vi "浊度电极校准.vi"() -> ()   [LabVIEW 2016, in "斯坦道多参数.lvlib"]
uses:
  <vilib>/Utility/miscctls.llb/LVPointTypeDef.ctl
  <vilib>/Utility/miscctls.llb/LVPositionTypeDef.ctl
  <vilib>/Analysis/NI_AALBase.lvlib
panel:
  in  "刷新按钮":bool
  out "第三点信号值":dbl
  out "第二点信号值":dbl
  out "第一点信号值":dbl
  out "温度":dbl format="%#.2f"
  out "通讯状态":string
  out "电极状态标志":u16(ring) items=["OK"=0, "第一点校正通过"=1, "第二点校正通过"=2, "悬浮物两点校准第一点校正通过"=11, "悬浮物两点校准第二点校正通过"=12, "浊度三点校正第一点校正通过"=31, "浊度三点校正第二点校正通过"=32, "浊度三点校正第三点校正通过"=33]
  out "第三点校准值":dbl
  out "标液3":dbl
  out "第二点校准值":dbl
  out "第一点校准值":dbl
  in  "校准停止":bool
  in  "校准启动":bool
  in  "校准模式":enum16{"两点校准", "单点校准", "三点校准"}(ring)
  out "最小值":sgl format="%#.2f"
  out "最大值":sgl format="%#.2f"
  out "波形图表":sgl(graph) caption="历史曲线"
  out "mean":dbl caption="均值" format="%#.2f"
  out "standard deviation":dbl caption="标准差" format="%#.2f"
  out "变异系数":dbl format="%#.6f"
  out "测量值":dbl format="%#.2f"
  out "提示":string
  out "标液2":dbl
  out "标液1":dbl
  out "信号值":dbl format="%#.2f"
  out "偏移值补偿":dbl caption="浊度偏移修正值" format="%#.2f"
  out "电极斜率":dbl format="%#.6f"
  out "电极零点":dbl format="%#.6f"
  # "浊度电极设定"
  # "℃"
  # "NTU"
  # "%"
  # "NTU"
  # "请选择校准模式:"
  # "NTU"
  # "NTU"
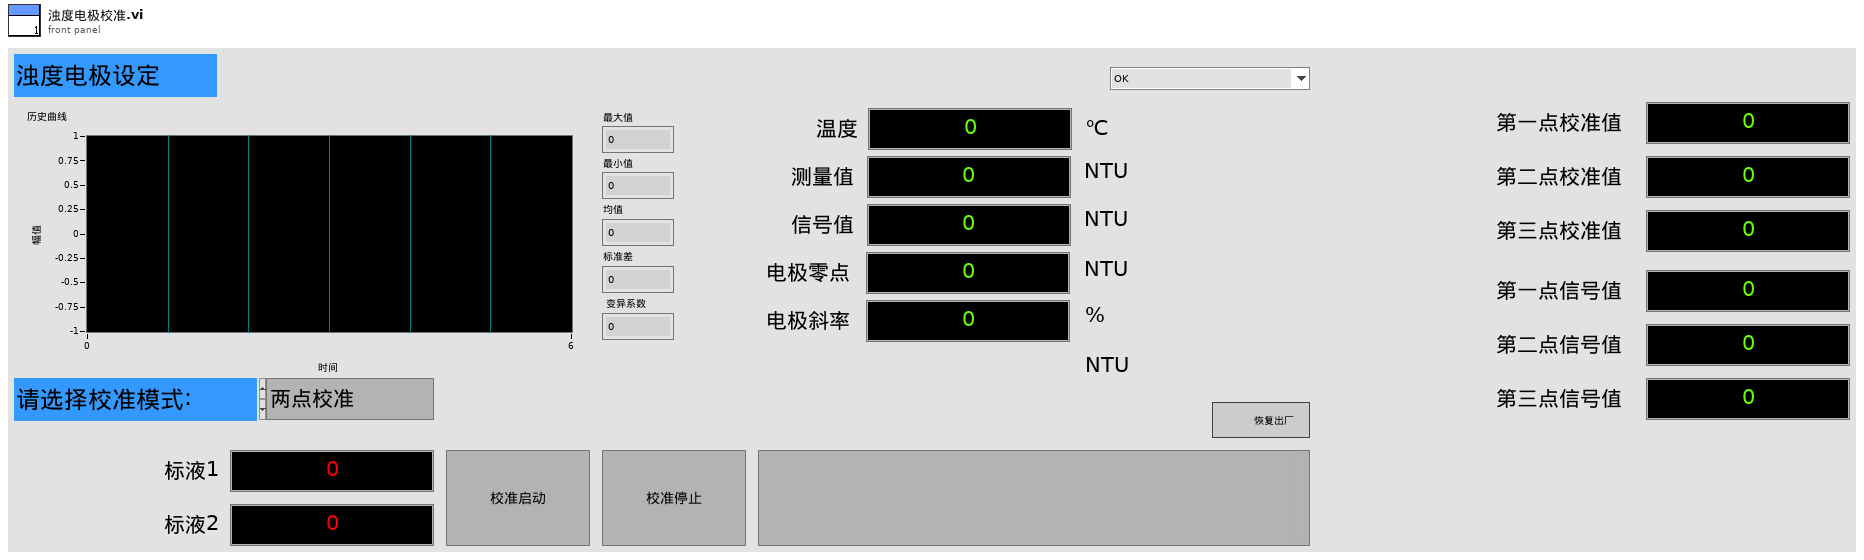
[diagram p1: front panel]
types:
  T1 = typedef "LVPointTypeDef.ctl" = cluster{"Horizontal":i16, "Vertical":i16}
  T2 = cluster{"电极状态标志":u16, "电极型号标志":u16, "浊度测量值":sgl, "温度测量值":sgl, "浊度信号值":sgl, "浊度偏移修正值":sgl, "温度偏移修正值":sgl, "手动温度补偿值":sgl, "浊度电极零点":sgl, "浊度电极斜率":sgl, "第1点标准值记录":sgl, "第1点信号值记录":sgl, "第1点温度值记录":sgl, "第2点标准值记录":sgl, "第2点信号值记录":sgl, "第2点温度值记录":sgl, "命令滤波设定":u16, "温度模式":enum16{"ATC", "MTC"}, "生产批次":u16, "电极序号":u16, "串口地址":u16, "串口波特率":enum16{"9600", "19200", "115200"}, "串口校验位":enum16{"NONE", "ODD", "EVEN"}, "串口停止位":enum16{"1bit", "2bit"}, "第一点标准值":sgl, "第二点标准值":sgl, "第三点标准值":sgl}
  T3 = typedef "LVPositionTypeDef.ctl" = cluster{"Left":i32, "Top":i32}
  T4 = enum8{"Enabled", "Disabled", "Disabled and Grayed Out"}
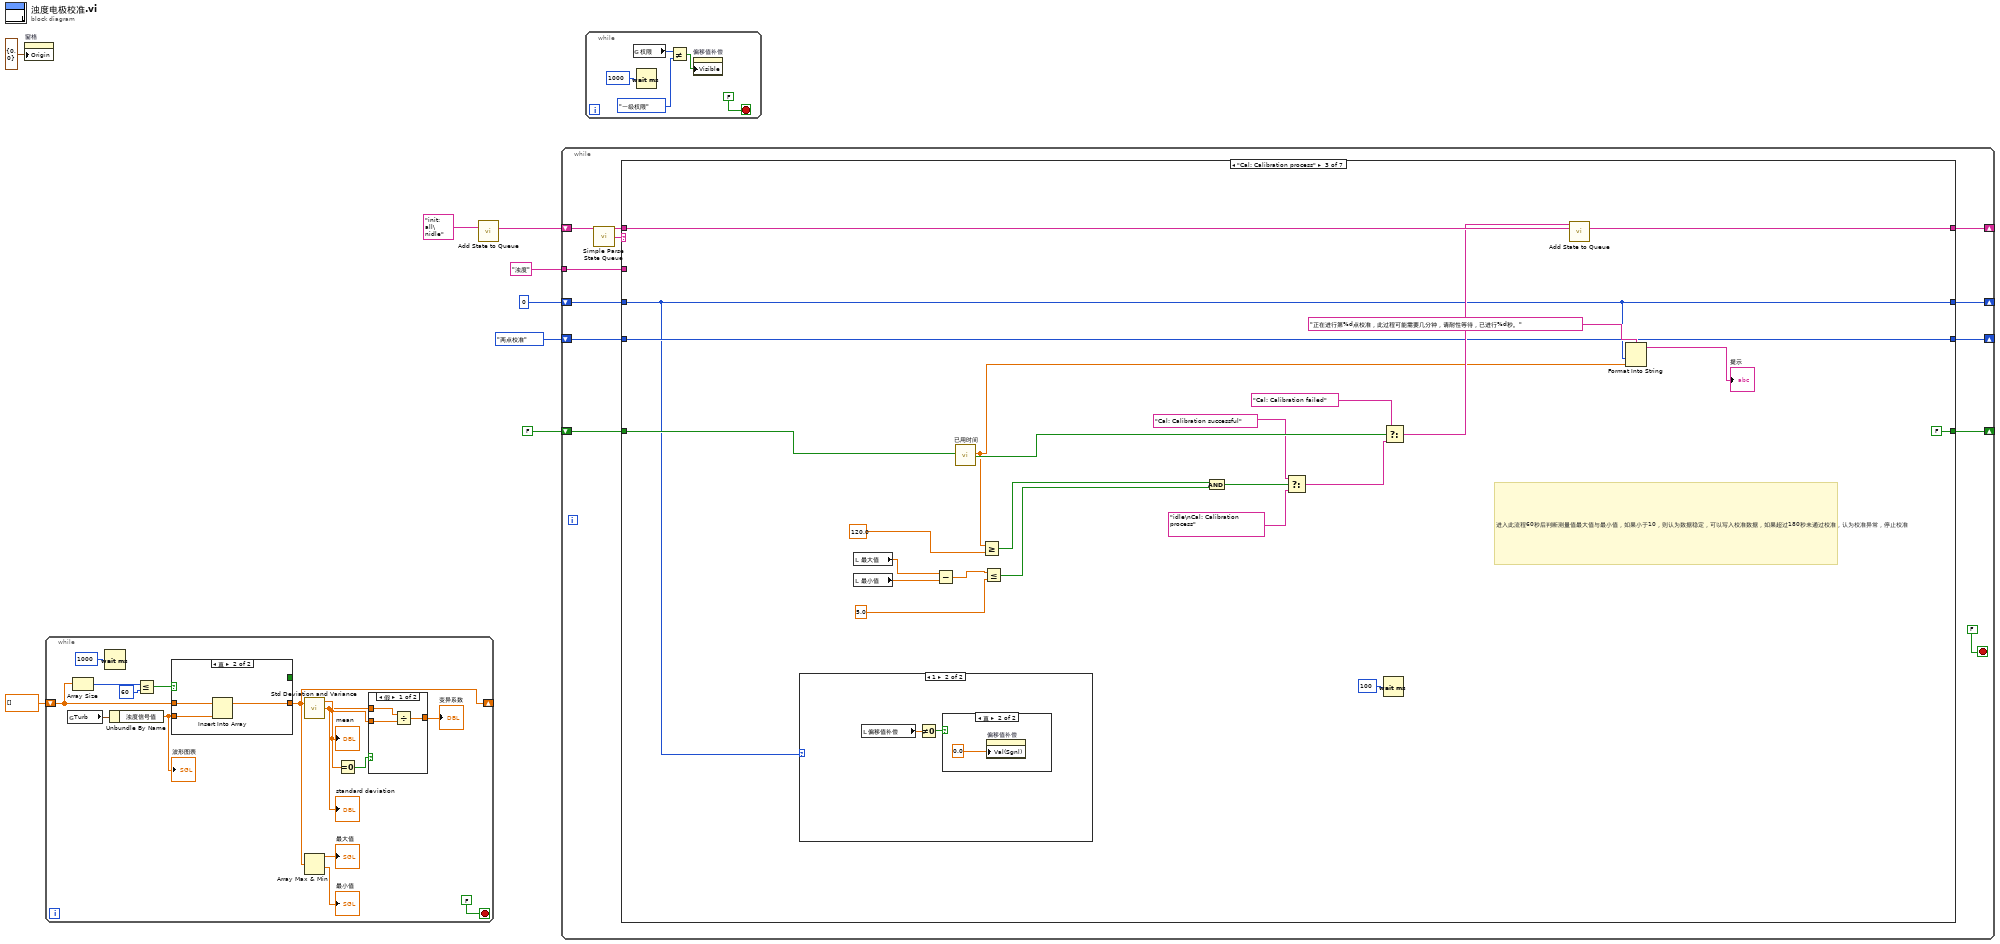
[diagram p0: block diagram]
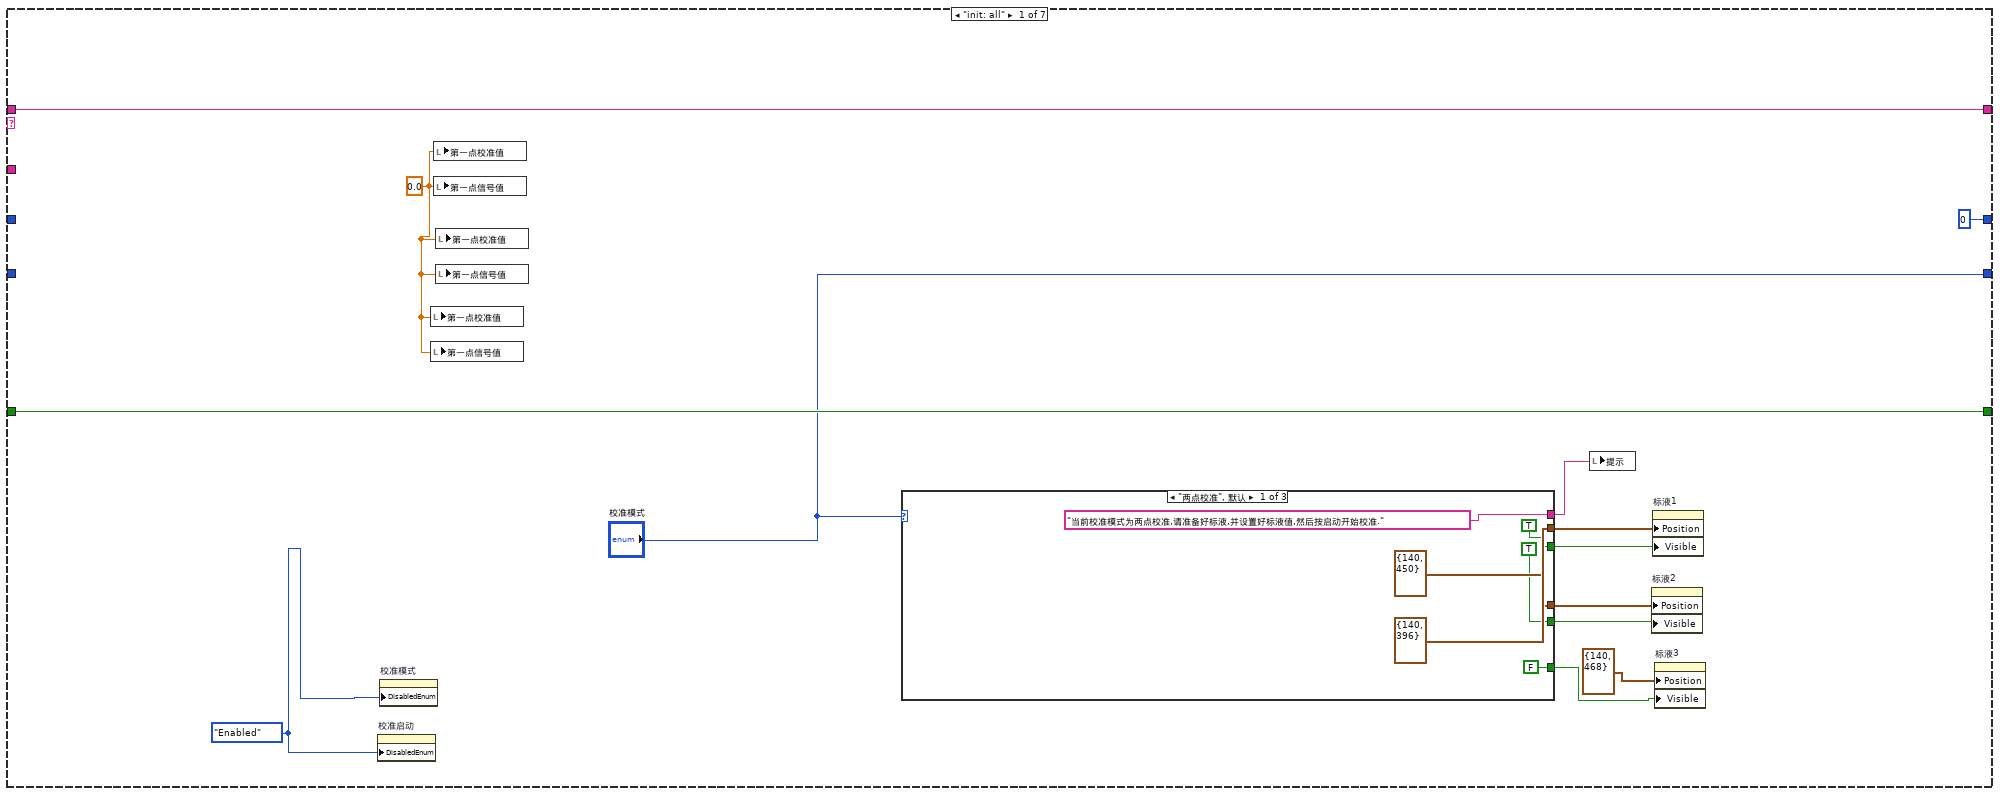
[diagram p2: hidden frame]
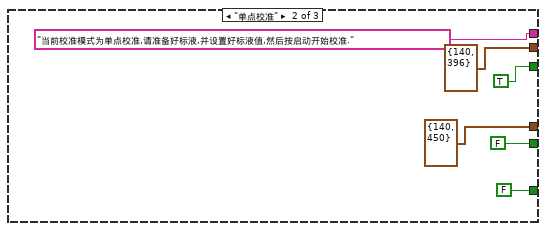
[diagram p3: hidden frame]
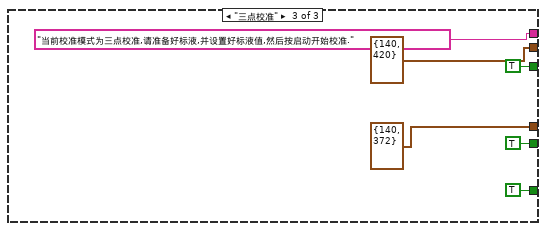
[diagram p4: hidden frame]
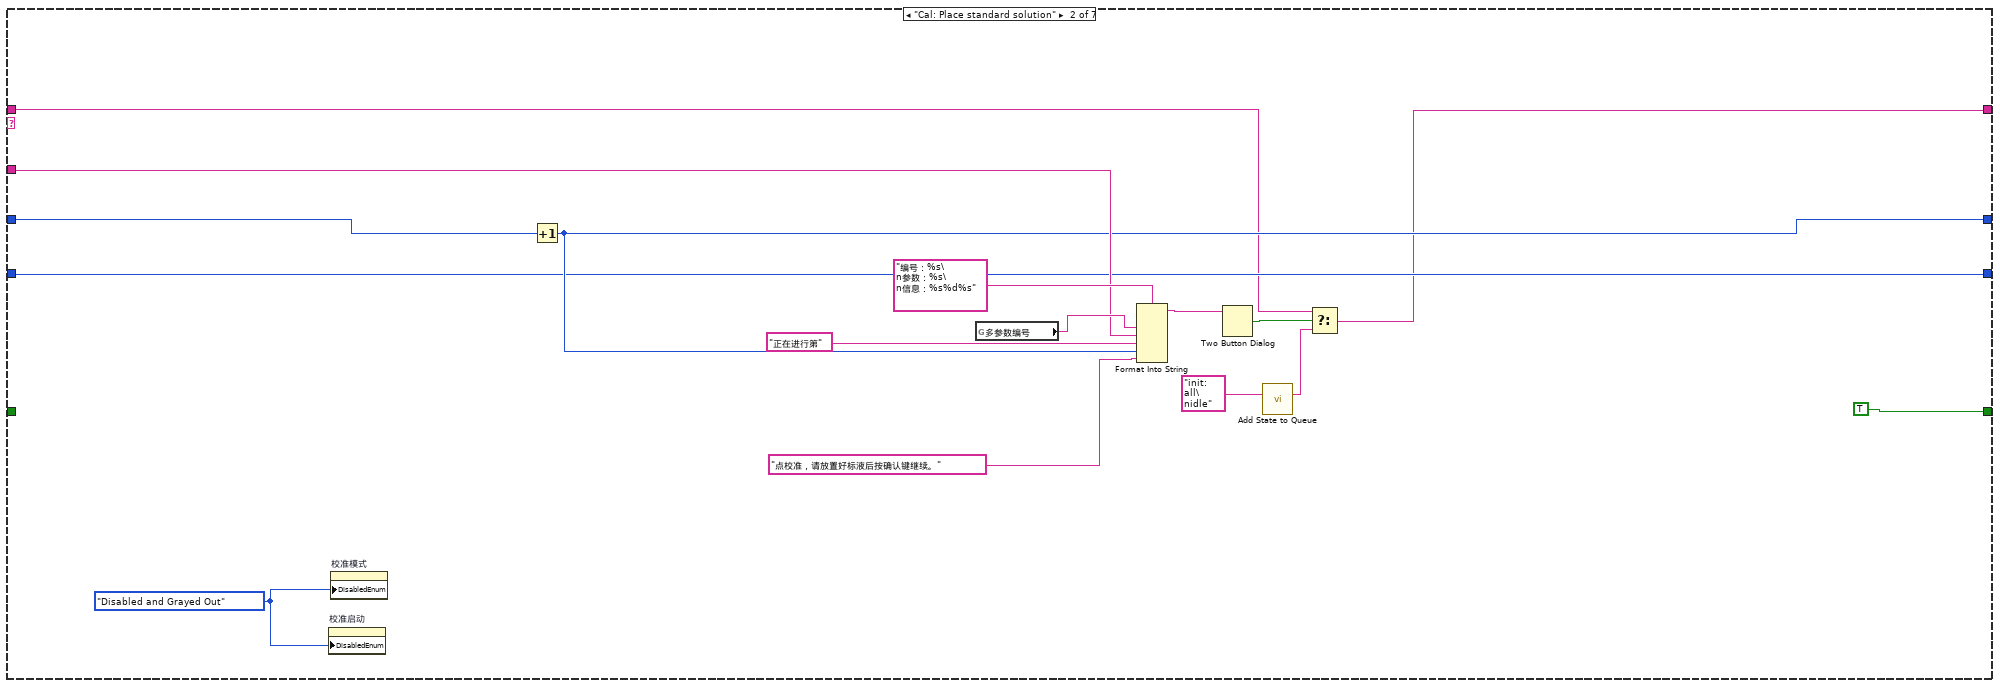
[diagram p5: hidden frame]
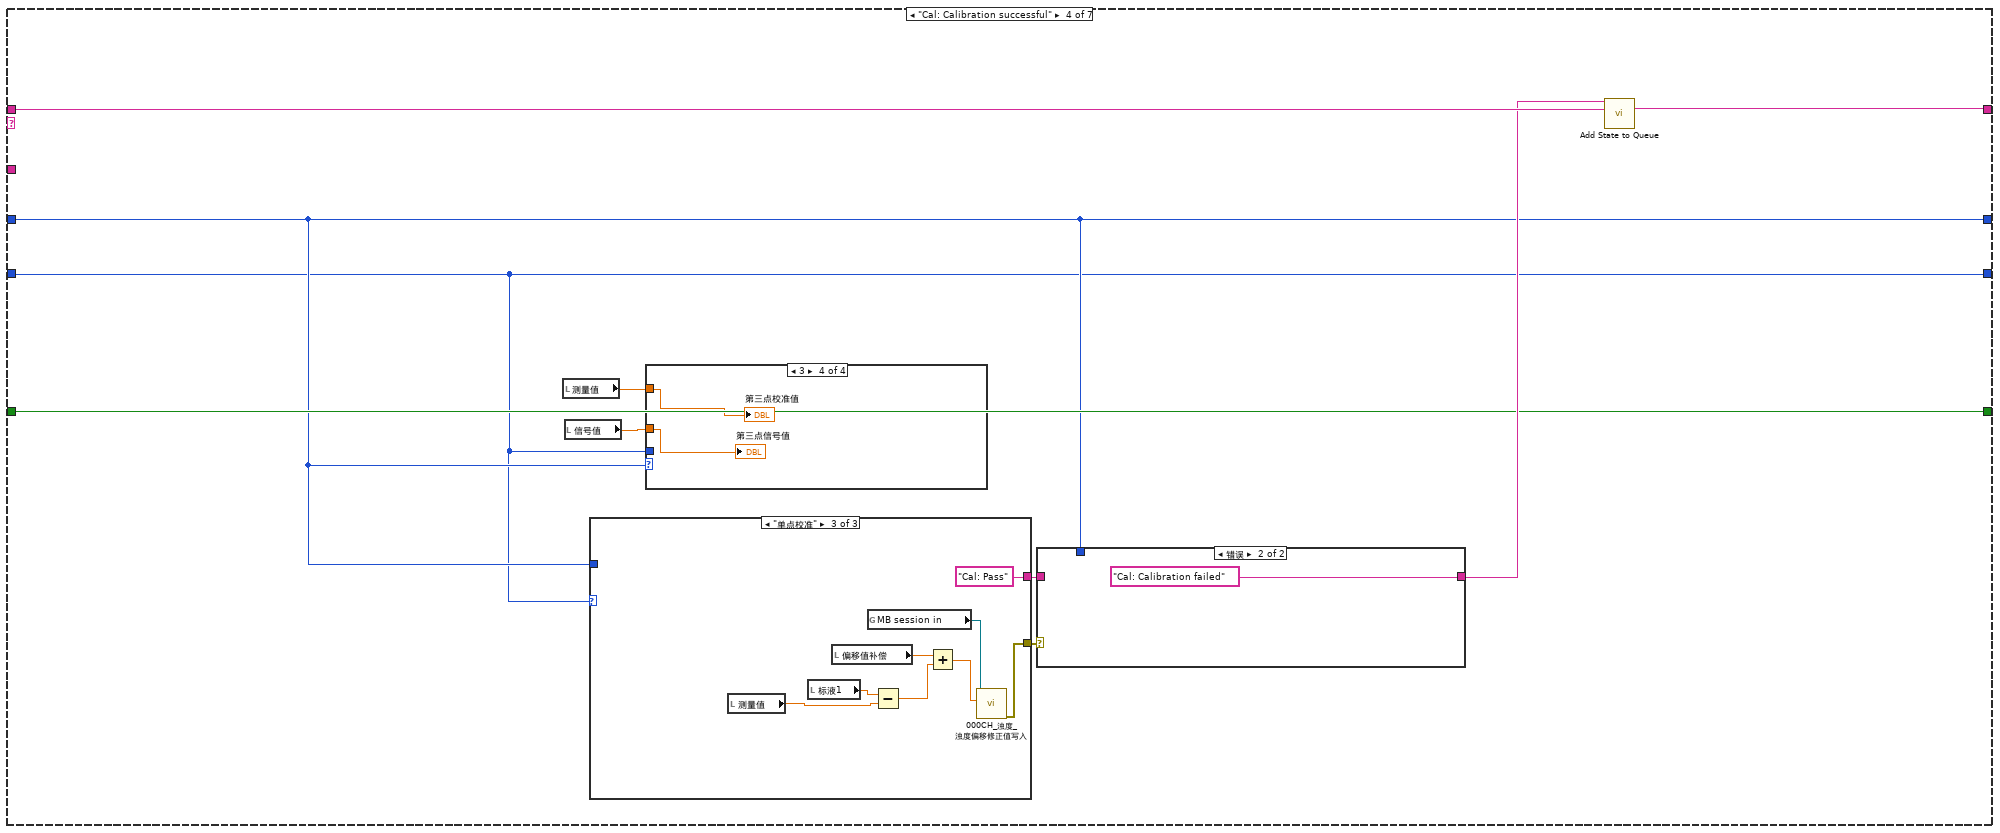
[diagram p8: hidden frame]
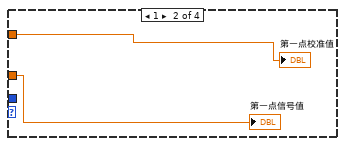
[diagram p10: hidden frame]
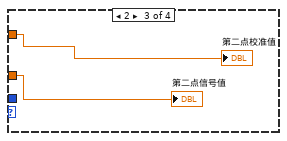
[diagram p11: hidden frame]
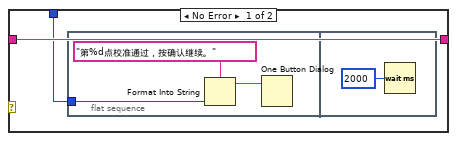
[diagram p12: hidden frame]
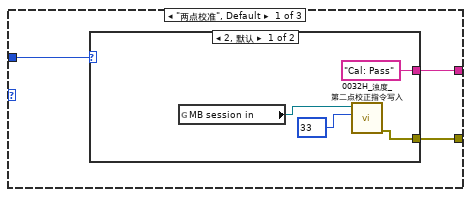
[diagram p13: hidden frame]
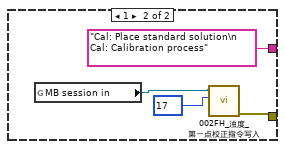
[diagram p14: hidden frame]
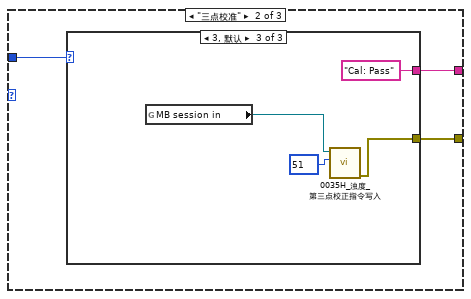
[diagram p15: hidden frame]
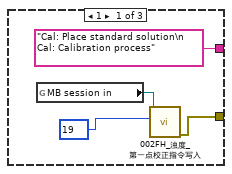
[diagram p16: hidden frame]
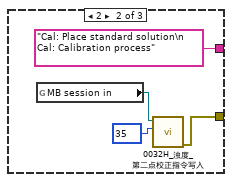
[diagram p17: hidden frame]
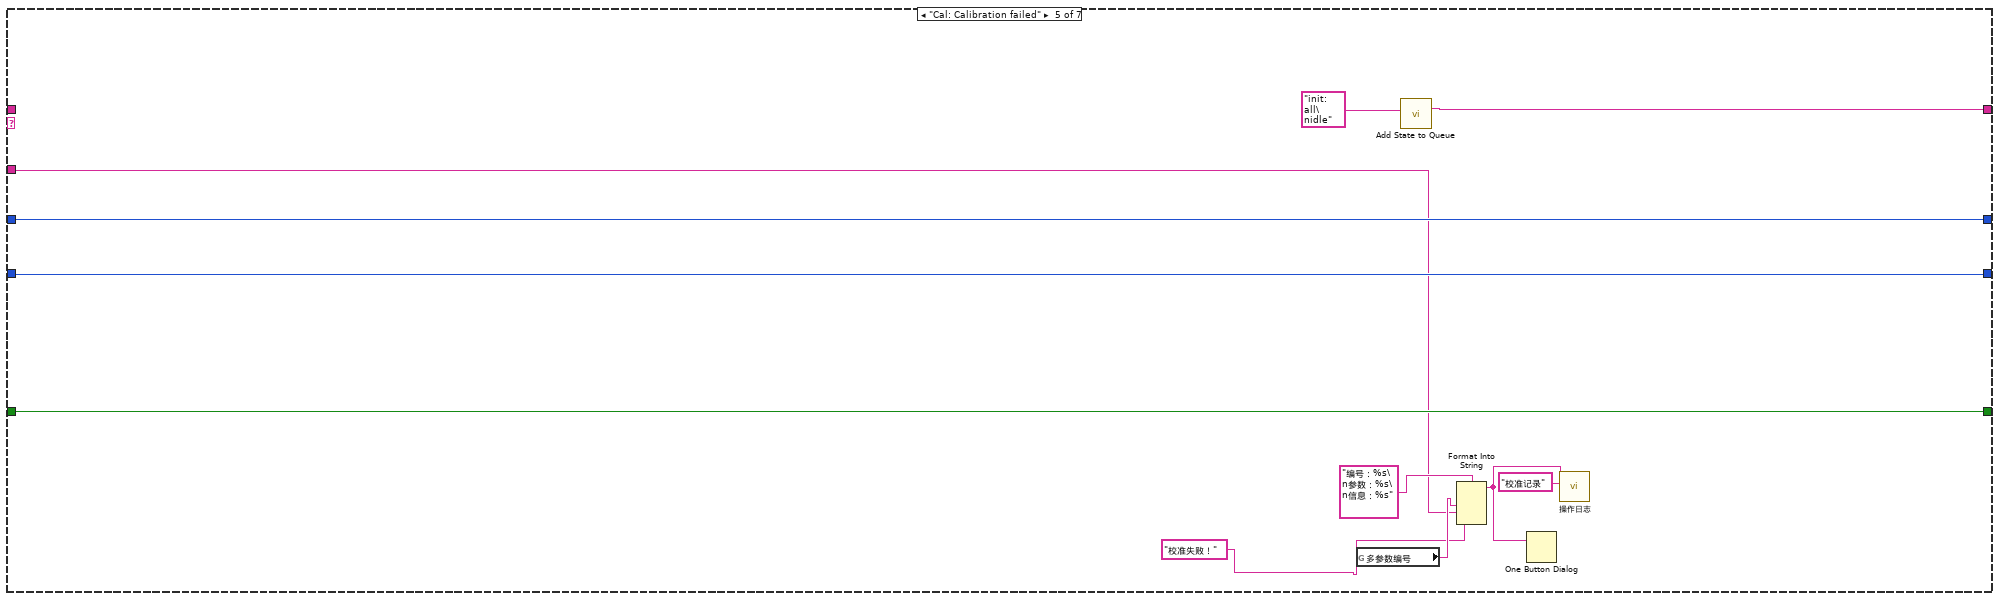
[diagram p18: hidden frame]
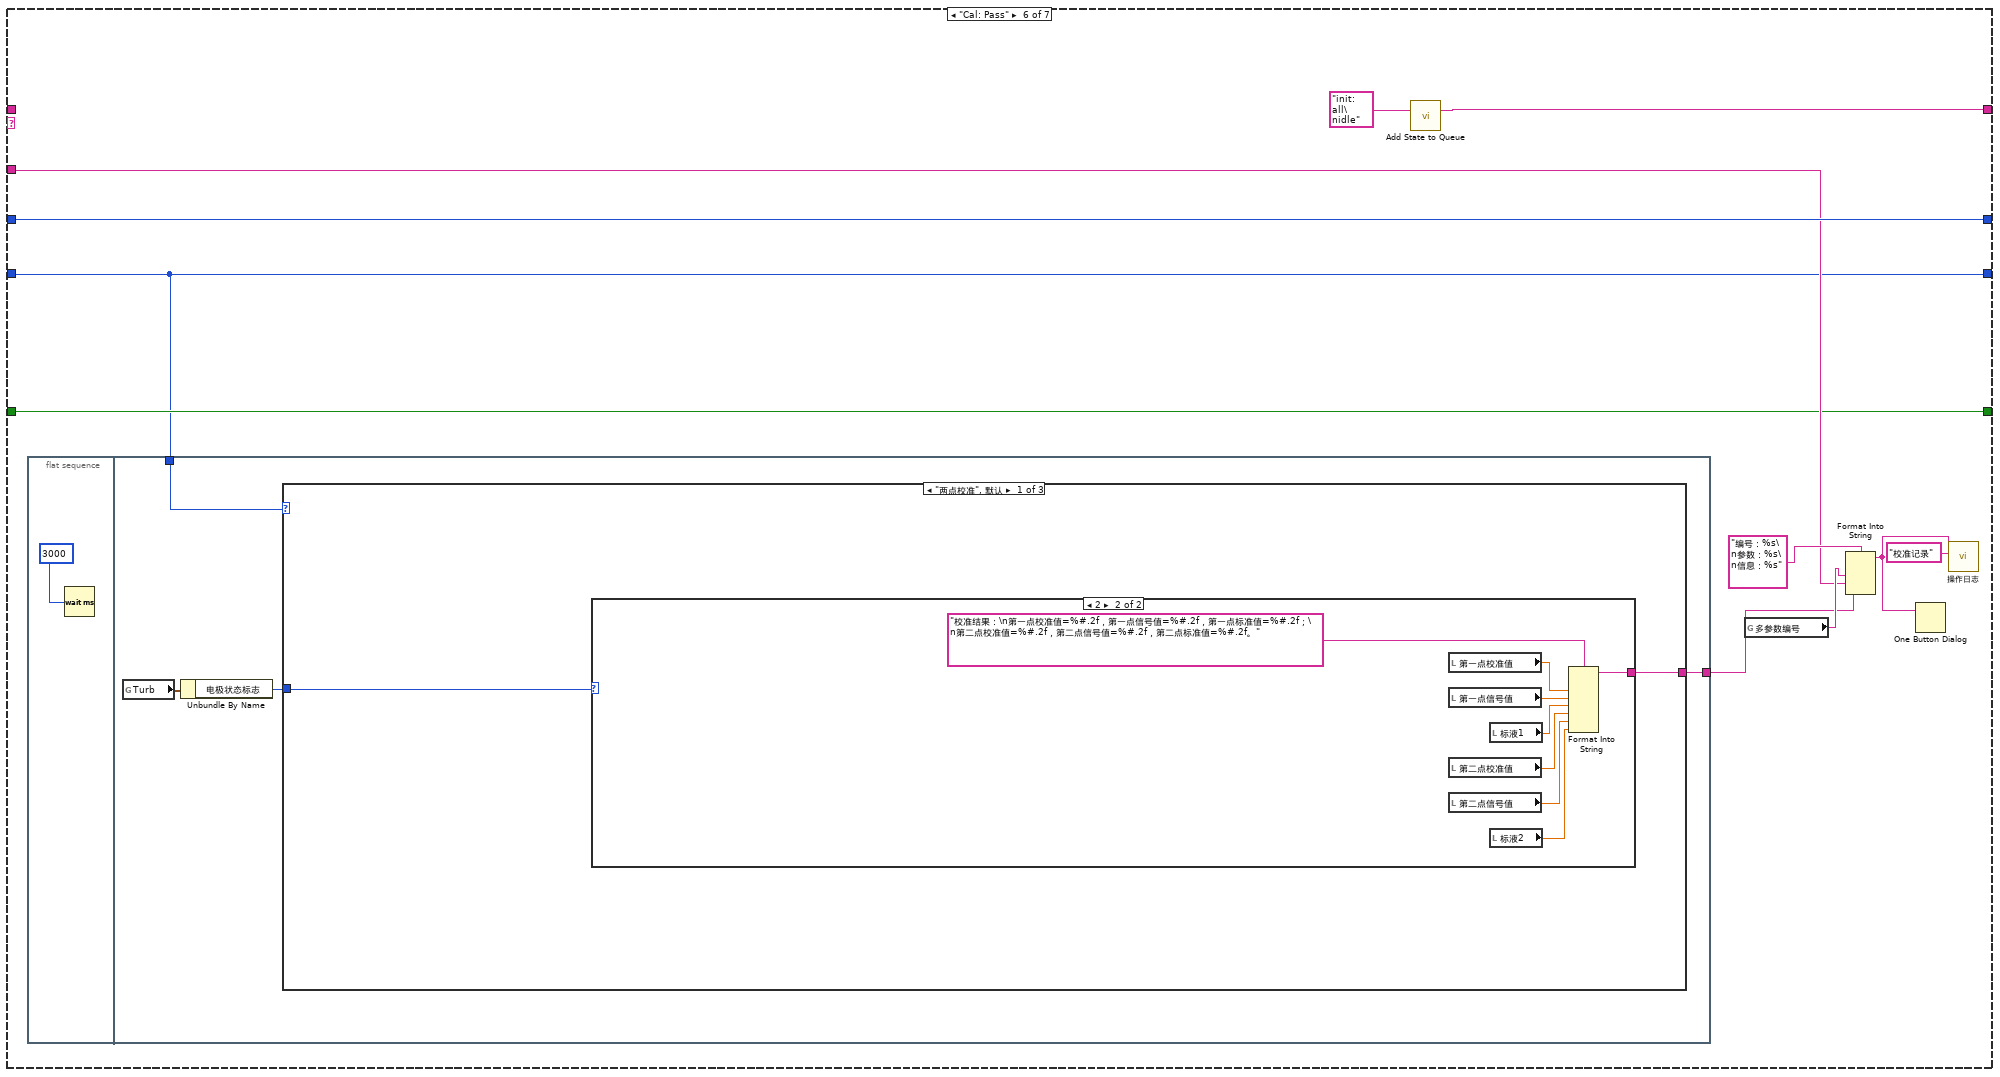
[diagram p19: hidden frame]
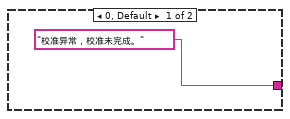
[diagram p20: hidden frame]
diagram:
  n1 = property on="窗格" class="Pane"("Origin"=T1 {"Horizontal"=0, "Vertical"=0} ("原点")) -> ()  [unwired: 2 in, 2 out]
  n2 = while {
    shift-right: [w12] -> _
    shift-left: sgl[] [] -> [w19]
    stop <- FALSE stop-if-true
    n3 = global read "国弘过程全局变量.vi" "Turb"() -> (w13:T2)
    n4 = Array Size(array=w19) -> (size(s)=w21:i32)
    n5 = Wait (ms)(milliseconds to wait=u32 1000 ("等待时间（毫秒）")) -> ()  [unwired: 1 out]
    n6 = Unbundle By Name(w13) -> ("浊度信号值"=w9:sgl)
    "波形图表" <- w9
    n7 = Less Or Equal?(x=w21, y=60) -> (x <= y?=w20:bool)
    n8 = case shown="真" w20 {
      tunnel: w19 -> [w32 w35]
      tunnel: w9 -> [w30 w34]
      tunnel: [w28 w33] -> w12
      tunnel: [TRUE _] -> _
      frame False {
        n9 = Replace Array Subset(array=w32, new element=w30) -> (w31:sgl[])  [unwired: 1 in]
        n10 = Rotate 1D Array(1:w31, 2:-1 ("n")) -> (0:w28:sgl[])
      }
      frame True {
        n11 = Insert Into Array(array=w35, new element=w34) -> (w33:sgl[])  [unwired: 1 in]
      }
    }
    n12 = call <vilib>:"Std Deviation and Variance.vi"("X"=w12) -> ("mean"=w17:dbl, "standard deviation"=w16:dbl)  [unwired: 1 in, 1 out]
    "mean" <- w17
    "standard deviation" <- w16
    n13 = Array Max & Min(array=w12) -> (max value=→"最大值":sgl, min value=→"最小值":sgl)  [unwired: 2 out]
    n14 = Equal To 0?(x=w17) -> (x = 0?=w18:bool)
    n15 = case shown="假" w18 {
      tunnel: w16 -> [w26 _]
      tunnel: [w25 _] -> w15
      tunnel: w17 -> [w24 _]
      frame False {
        n16 = Divide(x=w26, y=w24) -> (x/y=w25:dbl)
      }
      frame True {
      }
    }
    "变异系数" <- w15
  }
  n17 = call "Add State to Queue.vi"("State(s) In (\"\")"="init: all\nidle" ("State(s) In (\"\")")) -> ("States Out"=w5:string)  [unwired: 14 in]
  n18 = while {
    shift-right: [w43] -> _
    shift-left: w5 -> [w47]
    shift-right: [w40] -> _
    shift-left: 0 -> [w42]
    tunnel: "浊度" ("State(s) In (\"\")") -> [w41]
    shift-right: [w38] -> _
    shift-left: enum16{"两点校准", "单点校准", "三点校准"}."两点校准" ("校准模式") -> [w39]
    shift-right: [w36] -> _
    shift-left: FALSE -> [w37]
    stop <- FALSE stop-if-true
    n19 = call "Simple Parse State Queue.vi"("State Queue"=w47) -> ("Remain States"=w44:string, "Next State"=w45:string)  [unwired: 13 in]
    n20 = case shown="\"Cal: Calibration process\"" w45 {
      tunnel: w44 -> [w60 w81 w113 w129 _ _ w242]
      tunnel: [w60 w80 w112 w128 w186 w190 w241] -> w43
      tunnel: w42 -> [_ w90 w97 w123 w189 w200 w239]
      tunnel: w41 -> [_ w91 _ _ w179 w196 _]
      tunnel: [0 w88 w97 w123 w189 w200 w240] -> w40
      tunnel: w39 -> [_ w87 w98 w122 w188 w192 w238]
      tunnel: ["校准模式" w87 w98 w122 w188 w192 w238] -> w38
      tunnel: w37 -> [w57 _ w100 w124 w187 w195 w236]
      tunnel: [w57 TRUE FALSE w124 w187 w195 w236] -> w36
      frame "init: all" {
        w55 = T4."Enabled" ("禁用")
        w56 = 0.0 ("第一点校准值")
        n21 = property on="校准启动" class="Bool"("DisabledEnum"=w55) -> ()  [unwired: 2 in, 2 out]
        n22 = property on="校准模式" class="Enum (严格)"("DisabledEnum"=w55) -> ()  [unwired: 2 in, 2 out]
        n23 = local write "第一点校准值"(w56) -> ()
        n24 = local write "第一点信号值"(w56) -> ()
        n25 = local write "第一点校准值"(w56) -> ()
        n26 = local write "第一点信号值"(w56) -> ()
        n27 = local write "第一点校准值"(w56) -> ()
        n28 = local write "第一点信号值"(w56) -> ()
        n29 = case shown="\"两点校准\", 默认" "校准模式" {
          tunnel: ["当前校准模式为两点校准,请准备好标液,并设置好标液值,然后按启动开始校准." ("提示") "当前校准模式为单点校准,请准备好标液,并设置好标液值,然后按启动开始校准." ("提示") "当前校准模式为三点校准,请准备好标液,并设置好标液值,然后按启动开始校准." ("提示")] -> w59
          tunnel: [T3 {"Left"=140, "Top"=396} ("位置") T3 {"Left"=140, "Top"=396} ("位置") T3 {"Left"=140, "Top"=420} ("位置 2")] -> w53
          tunnel: [TRUE ("可见") TRUE ("可见") TRUE ("可见")] -> w52
          tunnel: [FALSE ("可见") FALSE ("可见") TRUE ("可见")] -> w50
          tunnel: [TRUE ("可见") FALSE ("可见") TRUE ("可见")] -> w49
          tunnel: [T3 {"Left"=140, "Top"=450} ("位置 2") T3 {"Left"=140, "Top"=450} ("位置 2") T3 {"Left"=140, "Top"=372} ("位置")] -> w48
          frame "两点校准", Default {
          }
          frame "单点校准" {
          }
          frame "三点校准" {
          }
        }
        n30 = local write "提示"(w59) -> ()
        n31 = property on="标液2" class="DigNum (严格)"("Position"=w48, "Visible"=w49) -> ()  [unwired: 2 in, 2 out]
        n32 = property on="标液1" class="DigNum (严格)"("Position"=w53, "Visible"=w52) -> ()  [unwired: 2 in, 2 out]
        n33 = property on="标液3" class="DigNum (严格)"("Position"=T3 {"Left"=140, "Top"=468} ("位置 3"), "Visible"=w50) -> ()  [unwired: 2 in, 2 out]
      }
      frame "Cal: Place standard solution" {
        w79 = T4."Disabled and Grayed Out" ("禁用")
        n34 = property on="校准启动" class="Bool"("DisabledEnum"=w79) -> ()  [unwired: 2 in, 2 out]
        n35 = property on="校准模式" class="Enum (严格)"("DisabledEnum"=w79) -> ()  [unwired: 2 in, 2 out]
        n36 = Increment(x=w90) -> (x+1=w88:i32)
        n37 = global read "多参数全局变量.vi" "多参数编号"() -> (w93:string)
        n38 = Format Into String(format string="编号：%s\n参数：%s\n信息：%s%d%s" ("格式字符串"), w93, w91, "正在进行第" ("消息"), w88, "点校准，请放置好标液后按确认键继续。" ("消息")) -> (resulting string=w85:string)  [unwired: 2 in, 1 out]
        n39 = Two Button Dialog(message=w85) -> (T button?=w84:bool)  [unwired: 2 in]
        n40 = call "Add State to Queue.vi"("State(s) In (\"\")"="init: all\nidle" ("State(s) In (\"\")")) -> ("States Out"=w82:string)  [unwired: 14 in]
        n41 = Select(t=w81, s=w84, f=w82) -> (s? t:f=w80:string)
      }
      frame "Cal: Calibration process" {
        # "进入此流程60秒后判断测量值最大值与最小值，如果小于10，则认为数据稳定，可以写入校准数据，如果超过180秒未通过校准，认为校准异常，停止校准"
        n42 = case shown="1" w97 {
          frame 0, Default {
          }
          frame 1 {
            n43 = local read "偏移值补偿"() -> (w119:dbl)
            n44 = Not Equal To 0?(x=w119) -> (x != 0?=w120:bool)
            n45 = case shown="真" w120 {
              frame False {
              }
              frame True {
                n46 = property on="偏移值补偿" class="DigNum (严格)"("Val(Sgnl)"=0.0 ("值(信号)")) -> ()  [unwired: 2 in, 2 out]
              }
            }
          }
        }
        n47 = local read "最大值"() -> (w117:sgl)
        n48 = local read "最小值"() -> (w116:sgl)
        n49 = Subtract(x=w117, y=w116) -> (x-y=w118:sgl)
        n50 = call "已用时间"("Reset"=w100) -> ("Elapsed Time (s)"=w96:dbl, "Time has Elapsed"=w114:bool)  [unwired: 11 in, 6 out]
        n51 = Greater Or Equal?(x=w96, y=120.0) -> (x >= y?=w109:bool)
        n52 = Less Or Equal?(x=w118, y=5.0) -> (x <= y?=w105:bool)
        n53 = And(x=w109, y=w105) -> (x .and. y?=w106:bool)
        n54 = Select(t="Cal: Calibration successful" ("State(s) In (\"\")"), s=w106, f="idle\nCal: Calibration process" ("State(s) In (\"\")")) -> (s? t:f=w104:string)
        n55 = Wait (ms)(milliseconds to wait=u32 100 ("等待时间（毫秒）")) -> ()  [unwired: 1 out]
        n56 = Select(t="Cal: Calibration failed" ("State(s) In (\"\")"), s=w114, f=w104) -> (s? t:f=w103:string)
        n57 = call "Add State to Queue.vi"("State(s) In Front (\"\")"=w103, "State(s) In (\"\")"=w113) -> ("States Out"=w112:string)  [unwired: 13 in]
        n58 = Format Into String(format string="正在进行第%d点校准，此过程可能需要几分钟，请耐性等待，已进行%d秒。" ("格式字符串"), w97, w96) -> (resulting string=→"提示":string)  [unwired: 2 in, 1 out]
      }
      frame "Cal: Calibration successful" {
        n59 = local read "测量值"() -> (w125:dbl)
        n60 = local read "信号值"() -> (w126:dbl)
        n61 = case shown="\"单点校准\"" w122 {
          tunnel: [w147 w158 w171] -> w131
          tunnel: [w146 w156 "Cal: Pass" ("State(s) In (\"\")")] -> w130
          tunnel: w123 -> [w145 w157 _]
          frame "两点校准", Default {
            n62 = case shown="2, 默认" w145 {
              tunnel: [w150 w154] -> w147
              tunnel: ["Cal: Pass" ("State(s) In (\"\")") "Cal: Place standard solution\n Cal: Calibration process" ("State(s) In (\"\")")] -> w146
              frame 2, Default {
                n63 = global read "多参数全局变量.vi" "MB session in"() -> (w149:refnum<class "MB_Master.lvclass">)
                n64 = call "0032H_浊度_第二点校正指令写入.vi"("数值"=u16 33, "MB session in"=w149) -> ("error out"=w150:errorcluster)  [unwired: 8 in, 1 out]
              }
              frame 1 {
                n65 = global read "多参数全局变量.vi" "MB session in"() -> (w153:refnum<class "MB_Master.lvclass">)
                n66 = call "002FH_浊度_第一点校正指令写入.vi"("数值"=u16 17, "MB session in"=w153) -> ("error out"=w154:errorcluster)  [unwired: 8 in, 1 out]
              }
            }
          }
          frame "三点校准" {
            n67 = case shown="3, 默认" w157 {
              tunnel: [w161 w164 w168] -> w158
              tunnel: ["Cal: Place standard solution\n Cal: Calibration process" ("State(s) In (\"\")") "Cal: Place standard solution\n Cal: Calibration process" ("State(s) In (\"\")") "Cal: Pass" ("State(s) In (\"\")")] -> w156
              frame 1 {
                n68 = global read "多参数全局变量.vi" "MB session in"() -> (w160:refnum<class "MB_Master.lvclass">)
                n69 = call "002FH_浊度_第一点校正指令写入.vi"("数值"=u16 19, "MB session in"=w160) -> ("error out"=w161:errorcluster)  [unwired: 8 in, 1 out]
              }
              frame 2 {
                n70 = global read "多参数全局变量.vi" "MB session in"() -> (w163:refnum<class "MB_Master.lvclass">)
                n71 = call "0032H_浊度_第二点校正指令写入.vi"("数值"=u16 35, "MB session in"=w163) -> ("error out"=w164:errorcluster)  [unwired: 8 in, 1 out]
              }
              frame 3, Default {
                n72 = global read "多参数全局变量.vi" "MB session in"() -> (w167:refnum<class "MB_Master.lvclass">)
                n73 = call "0035H_浊度_第三点校正指令写入.vi"("数值"=u16 51, "MB session in"=w167) -> ("error out"=w168:errorcluster)  [unwired: 8 in, 1 out]
              }
            }
          }
          frame "单点校准" {
            n74 = local read "测量值"() -> (w174:dbl)
            n75 = local read "标液1"() -> (w178:dbl)
            n76 = local read "偏移值补偿"() -> (w176:dbl)
            n77 = global read "多参数全局变量.vi" "MB session in"() -> (w173:refnum<class "MB_Master.lvclass">)
            n78 = Subtract(x=w178, y=w174) -> (x-y=w177:dbl)
            n79 = Add(x=w176, y=w177) -> (x+y=w172:dbl)
            n80 = call "000CH_浊度_浊度偏移修正值写入.vi"("数值"=w172, "MB session in"=w173) -> ("error out"=w171:errorcluster)  [unwired: 8 in, 1 out]
          }
        }
        n81 = case shown="3" w123 {
          tunnel: w126 -> [_ w133 w135 w137]
          tunnel: w125 -> [_ w132 w134 w136]
          tunnel: w122 -> [_ _ _ _]
          frame 0, Default {
          }
          frame 1 {
            "第一点信号值" <- w133
            "第一点校准值" <- w132
          }
          frame 2 {
            "第二点信号值" <- w135
            "第二点校准值" <- w134
          }
          frame 3 {
            "第三点信号值" <- w137
            "第三点校准值" <- w136
          }
        }
        n82 = case shown="错误" w131 {
          tunnel: w130 -> [w139 _]
          tunnel: [w139 "Cal: Calibration failed" ("State(s) In (\"\")")] -> w127
          tunnel: w123 -> [w138 _]
          frame No Error {
            n83 = flat-sequence {
              tunnel: w138 -> [w140]
              frame #0 {
                n84 = Format Into String(format string="第%d点校准通过，按确认继续。" ("格式字符串"), w140) -> (resulting string=w142:string)  [unwired: 2 in, 1 out]
                n85 = One Button Dialog(message=w142) -> ()  [unwired: 1 in, 1 out]
              }
              frame #1 {
                n86 = Wait (ms)(milliseconds to wait=u32 2000 ("等待时间（毫秒）")) -> ()  [unwired: 1 out]
              }
            }
          }
          frame Error {
          }
        }
        n87 = call "Add State to Queue.vi"("State(s) In Front (\"\")"=w127, "State(s) In (\"\")"=w129) -> ("States Out"=w128:string)  [unwired: 13 in]
      }
      frame "Cal: Calibration failed" {
        n88 = global read "多参数全局变量.vi" "多参数编号"() -> (w182:string)
        n89 = call "Add State to Queue.vi"("State(s) In (\"\")"="init: all\nidle" ("State(s) In (\"\")")) -> ("States Out"=w186:string)  [unwired: 14 in]
        n90 = Format Into String(format string="编号：%s\n参数：%s\n信息：%s" ("格式字符串"), w182, w179, "校准失败！" ("消息")) -> (resulting string=w181:string)  [unwired: 2 in, 1 out]
        n91 = One Button Dialog(message=w181) -> ()  [unwired: 1 in, 1 out]
        n92 = call "操作日志.vi"("table"="校准记录", "日志信息"=w181) -> ()  [unwired: 9 in, 1 out]
      }
      frame "Cal: Pass" {
        n93 = flat-sequence {
          tunnel: [w203] -> w193
          tunnel: w192 -> [w202]
          frame #0 {
            n94 = Wait (ms)(milliseconds to wait=u32 3000 ("等待时间（毫秒）")) -> ()  [unwired: 1 out]
          }
          frame #1 {
            n95 = global read "国弘过程全局变量.vi" "Turb"() -> (w204:T2)
            n96 = Unbundle By Name(w204) -> ("电极状态标志"=w205:u16)
            n97 = case shown="\"两点校准\", 默认" w202 {
              tunnel: [w207 w218 w235] -> w203
              tunnel: w205 -> [w206 w217 _]
              frame "两点校准", Default {
                n98 = case shown="2" w206 {
                  tunnel: ["校准异常，校准未完成。" ("格式字符串") w216] -> w207
                  frame 0, Default {
                  }
                  frame 2 {
                    n99 = local read "第一点校准值"() -> (w214:dbl)
                    n100 = local read "第一点信号值"() -> (w215:dbl)
                    n101 = local read "第二点校准值"() -> (w211:dbl)
                    n102 = local read "第二点信号值"() -> (w210:dbl)
                    n103 = local read "标液1"() -> (w212:dbl)
                    n104 = local read "标液2"() -> (w209:dbl)
                    n105 = Format Into String(format string="校准结果：\n第一点校准值=%#.2f，第一点信号值=%#.2f，第一点标准值=%#.2f；\n第二点校准值=%#.2f，第二点信号值=%#.2f，第二点标准值=%#.2f。" ("提示"), w214, w215, w212, w211, w210, w209) -> (resulting string=w216:string)  [unwired: 2 in, 1 out]
                  }
                }
              }
              frame "三点校准" {
                n106 = case shown="33" w217 {
                  tunnel: ["校准异常，校准未完成。" ("格式字符串") w230] -> w218
                  frame 0, Default {
                  }
                  frame 33 {
                    n107 = local read "标液2"() -> (w221:dbl)
                    n108 = local read "标液1"() -> (w222:dbl)
                    n109 = local read "第一点校准值"() -> (w229:dbl)
                    n110 = local read "第一点信号值"() -> (w227:dbl)
                    n111 = local read "第二点校准值"() -> (w226:dbl)
                    n112 = local read "第二点信号值"() -> (w225:dbl)
                    n113 = local read "第三点校准值"() -> (w224:dbl)
                    n114 = local read "第三点信号值"() -> (w223:dbl)
                    n115 = local read "标液3"() -> (w220:dbl)
                    n116 = Format Into String(format string="校准结果：\n第一点校准值=%#.2f，第一点信号值=%#.2f，第一点标准值=%#.2f；\n第二点校准值=%#.2f，第二点信号值=%#.2f，第二点标准值=%#.2f；\n第三点校准值=%#.2f，第三点信号值=%#.2f，第三点标准值=%#.2f。" ("提示"), w229, w227, w222, w226, w225, w221, w224, w223, w220) -> (resulting string=w230:string)  [unwired: 2 in, 1 out]
                  }
                }
              }
              frame "单点校准" {
                n117 = local read "第一点校准值"() -> (w234:dbl)
                n118 = local read "第一点信号值"() -> (w232:dbl)
                n119 = local read "标液1"() -> (w231:dbl)
                n120 = Format Into String(format string="校准结果：\n校准值=%#.2f，信号值=%#.2f，标准值=%#.2f。" ("提示"), w234, w232, w231) -> (resulting string=w235:string)  [unwired: 2 in, 1 out]
              }
            }
          }
        }
        n121 = call "Add State to Queue.vi"("State(s) In (\"\")"="init: all\nidle" ("State(s) In (\"\")")) -> ("States Out"=w190:string)  [unwired: 14 in]
        n122 = global read "多参数全局变量.vi" "多参数编号"() -> (w197:string)
        n123 = Format Into String(format string="编号：%s\n参数：%s\n信息：%s" ("格式字符串"), w197, w196, w193) -> (resulting string=w194:string)  [unwired: 2 in, 1 out]
        n124 = One Button Dialog(message=w194) -> ()  [unwired: 1 in, 1 out]
        n125 = call "操作日志.vi"("table"="校准记录", "日志信息"=w194) -> ()  [unwired: 9 in, 1 out]
      }
      frame "idle", Default {
        n126 = event shown="[0] 超时" {
          selector: _ -> [_ _ _ _ _ _ _ _ _ _]
          dyn-events: _ -> [_ _ _ _ _ _ _ _ _ _]
          timeout: 10 -> [_ _ _ _ _ _ _ _ _ _]
          tunnel: [_ _ _ w276 w283 w289 w295 _ _ _] -> _
          tunnel: w242 -> [w260 w264 w267 w279 w280 w286 w292 w302 w308 _]
          tunnel: [w259 w263 w268 w278 w284 w290 w296 w301 w307 w310] -> w241
          tunnel: [w258 w261 w269 w277 w285 w291 w297 w300 w305 w311] -> w240
          tunnel: w239 -> [w258 w261 w269 w277 w285 w291 w297 w300 w305 w311]
          event Timeout {
            n127 = event-data() -> ()  [unwired: 1 in, 3 out]
            n128 = global read "国弘过程全局变量.vi" "Turb"() -> (w243:T2)
            n129 = Unbundle By Name(w243) -> ("电极状态标志"=→"电极状态标志":u16, "浊度电极零点"=→"电极零点":sgl, "浊度电极斜率"=→"电极斜率":sgl, "浊度偏移修正值"=→"偏移值补偿":sgl, "浊度信号值"=→"信号值":sgl, "第一点标准值"=→"标液1":sgl, "第二点标准值"=→"标液2":sgl, "浊度测量值"=→"测量值":sgl, "第三点标准值"=→"标液3":sgl, "温度测量值"=→"温度":sgl)  [unwired: 1 out]
            n130 = global read "多参数全局变量.vi" "浊度通讯状态"() -> (w255:bool)
            n131 = property on="通讯状态" class="Str"("Blinking"=TRUE ("闪烁"), "Text.BG Color"=u32 16711680, "Visible"=w255) -> ()  [unwired: 2 in, 2 out]
            n132 = call "Add State to Queue.vi"("State(s) In (\"\")"=w260) -> ("States Out"=w259:string)  [unwired: 14 in]
            "通讯状态" <- "通讯异常" ("当前串口")
          }
          event "校准模式": Value Change {
            n133 = event-data() -> ()  [unwired: 1 in, 6 out]
            n134 = call "Add State to Queue.vi"("State(s) In (\"\")"=w264, "State(s) At Back (\"\")"="init: all\nidle" ("State(s) In (\"\")")) -> ("States Out"=w263:string)  [unwired: 13 in]
          }
          event "偏移值补偿", "标液1", "标液2", "标液3": Mouse Down {
            n135 = event-data() -> ("CtlRef"=w266:refnum<vi>)  [unwired: 1 in, 7 out]
            n136 = property class="DigNum (严格)"(reference=w266) -> ("DisabledEnum"=w265:T4)  [unwired: 1 in, 2 out]
            n137 = case shown="\"Enabled\"" w265 {
              tunnel: w266 -> [w273 _]
              frame "Enabled" {
                n138 = property class="DigNum (严格)"(reference=w273) -> (reference out=w270:refnum<vi>, "Value"=w271:dbl)  [unwired: 1 in, 1 out]
                n139 = call "数字键盘.vi"("OldNumber"=w271) -> ("NewNumber"=w272:dbl)  [unwired: 1 in]
                n140 = property class="DigNum (严格)"(reference=w270, "Val(Sgnl)"=w272) -> ()  [unwired: 1 in, 2 out]
              }
              frame "Disabled", Default {
              }
            }
            n141 = call "Add State to Queue.vi"("State(s) In (\"\")"=w267) -> ("States Out"=w268:string)  [unwired: 14 in]
          }
          event "偏移值补偿": Value Change {
            n142 = event-data() -> ("NewVal"=w274:dbl)  [unwired: 1 in, 5 out]
            n143 = global read "多参数全局变量.vi" "MB session in"() -> (w275:refnum<class "MB_Master.lvclass">)
            n144 = call "000CH_浊度_浊度偏移修正值写入.vi"("数值"=w274, "MB session in"=w275) -> ("error out"=w276:errorcluster)  [unwired: 8 in, 1 out]
            n145 = call "Add State to Queue.vi"("State(s) In (\"\")"=w279) -> ("States Out"=w278:string)  [unwired: 14 in]
          }
          event "标液1": Value Change {
            n146 = event-data() -> ("NewVal"=w281:dbl)  [unwired: 1 in, 5 out]
            n147 = global read "多参数全局变量.vi" "MB session in"() -> (w282:refnum<class "MB_Master.lvclass">)
            n148 = call "0030H_浊度_第一点标准值写入.vi"("数值"=w281, "MB session in"=w282) -> ("error out"=w283:errorcluster)  [unwired: 8 in, 1 out]
            n149 = call "Add State to Queue.vi"("State(s) In (\"\")"=w280) -> ("States Out"=w284:string)  [unwired: 14 in]
          }
          event "标液2": Value Change {
            n150 = event-data() -> ("NewVal"=w287:dbl)  [unwired: 1 in, 5 out]
            n151 = global read "多参数全局变量.vi" "MB session in"() -> (w288:refnum<class "MB_Master.lvclass">)
            n152 = call "0033H_浊度_第二点标准值写入.vi"("数值"=w287, "MB session in"=w288) -> ("error out"=w289:errorcluster)  [unwired: 8 in, 1 out]
            n153 = call "Add State to Queue.vi"("State(s) In (\"\")"=w286) -> ("States Out"=w290:string)  [unwired: 14 in]
          }
          event "标液3": Value Change {
            n154 = event-data() -> ("NewVal"=w293:dbl)  [unwired: 1 in, 5 out]
            n155 = global read "多参数全局变量.vi" "MB session in"() -> (w294:refnum<class "MB_Master.lvclass">)
            n156 = call "0036H_浊度_第三点标准值写入.vi"("数值"=w293, "MB session in"=w294) -> ("error out"=w295:errorcluster)  [unwired: 8 in, 1 out]
            n157 = call "Add State to Queue.vi"("State(s) In (\"\")"=w292) -> ("States Out"=w296:string)  [unwired: 14 in]
          }
          event "刷新按钮": Value Change {
            n158 = event-data() -> ()  [unwired: 1 in, 6 out]
            n159 = call "Add State to Queue.vi"("State(s) In (\"\")"=w302) -> ("States Out"=w301:string)  [unwired: 14 in]
            n160 = Two Button Dialog(message="请再次确实是否恢复出厂设置！" ("消息")) -> (T button?=w299:bool)  [unwired: 2 in]
            n161 = case shown="真" w299 {
              frame False {
              }
              frame True {
                w303 = u16 33 items=["Factory Reset"=33] ("数值")
                n162 = global read "多参数全局变量.vi" "MB session in"() -> (w304:refnum<class "MB_Master.lvclass">)
                n163 = call "0026H_浊度_命令寄存器写入.vi"("数值"=w303, "MB session in"=w304) -> ()  [unwired: 8 in, 2 out]
              }
            }
          }
          event "校准启动": Value Change {
            n164 = event-data() -> ()  [unwired: 1 in, 6 out]
            n165 = call "Add State to Queue.vi"("State(s) In (\"\")"=w308, "State(s) At Back (\"\")"="init: all\nCal: Place standard solution\n Cal: Calibration process\nidle" ("State(s) In (\"\")")) -> ("States Out"=w307:string)  [unwired: 13 in]
          }
          event "校准停止": Value Change {
            n166 = event-data() -> ()  [unwired: 1 in, 6 out]
            n167 = call "Add State to Queue.vi"("State(s) In (\"\")"="init: all\nidle" ("State(s) In (\"\")")) -> ("States Out"=w310:string)  [unwired: 14 in]
          }
        }
      }
    }
  }
  n168 = while {
    stop <- FALSE stop-if-true
    n169 = global read "多参数全局变量.vi" "权限"() -> (w315:enum16{"一级权限", "二级权限", "三级权限"})
    n170 = Wait (ms)(milliseconds to wait=u32 1000 ("等待时间（毫秒）")) -> ()  [unwired: 1 out]
    n171 = Not Equal?(x=w315, y=enum16{"一级权限", "二级权限", "三级权限"}."一级权限") -> (x != y?=w313:bool)
    n172 = property on="偏移值补偿" class="DigNum (严格)"("Visible"=w313) -> ()  [unwired: 2 in, 2 out]
  }
